vi "intersecAreaQuad.vi"(8 "error in (no error)":errorcluster, 9 "Ball/Enemy\nPosition":dbl[](array[numeric]), 10 "Game":refnum<class "Game.lvclass">, 11 "Utilities in":refnum<class "Utilities.lvclass">) -> (0 "error out":errorcluster, 2 "Pos de Interseção":dbl[](array[numeric]) format="%#_13g", 3 "Utilities out":refnum<class "Utilities.lvclass">)   [LabVIEW 2018, in "Utilities.lvclass"]
uses:
  Utilities.lvclass
  Game_class/Game.lvclass
  Game_class/Game.lvclass/Game.ctl
  Game_class/Read FieldRef.vi
  Field_class/Field.lvclass
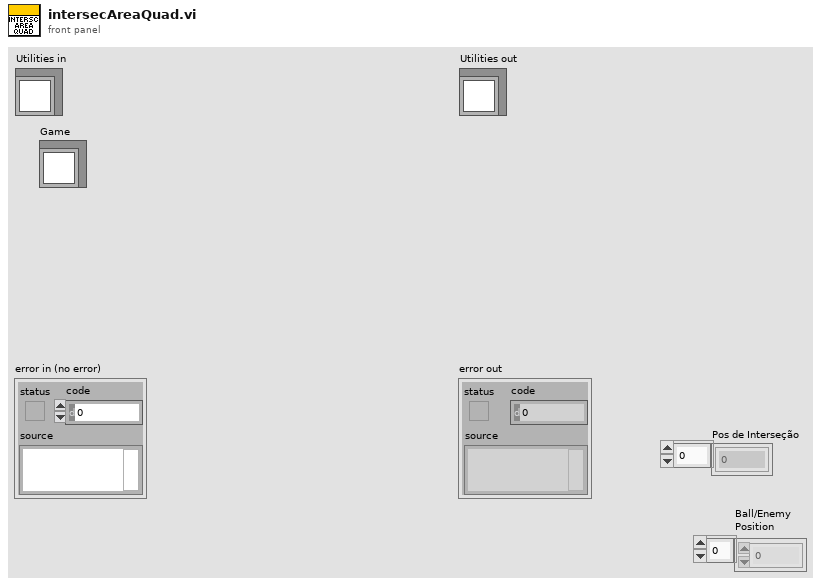
[diagram p1: front panel]
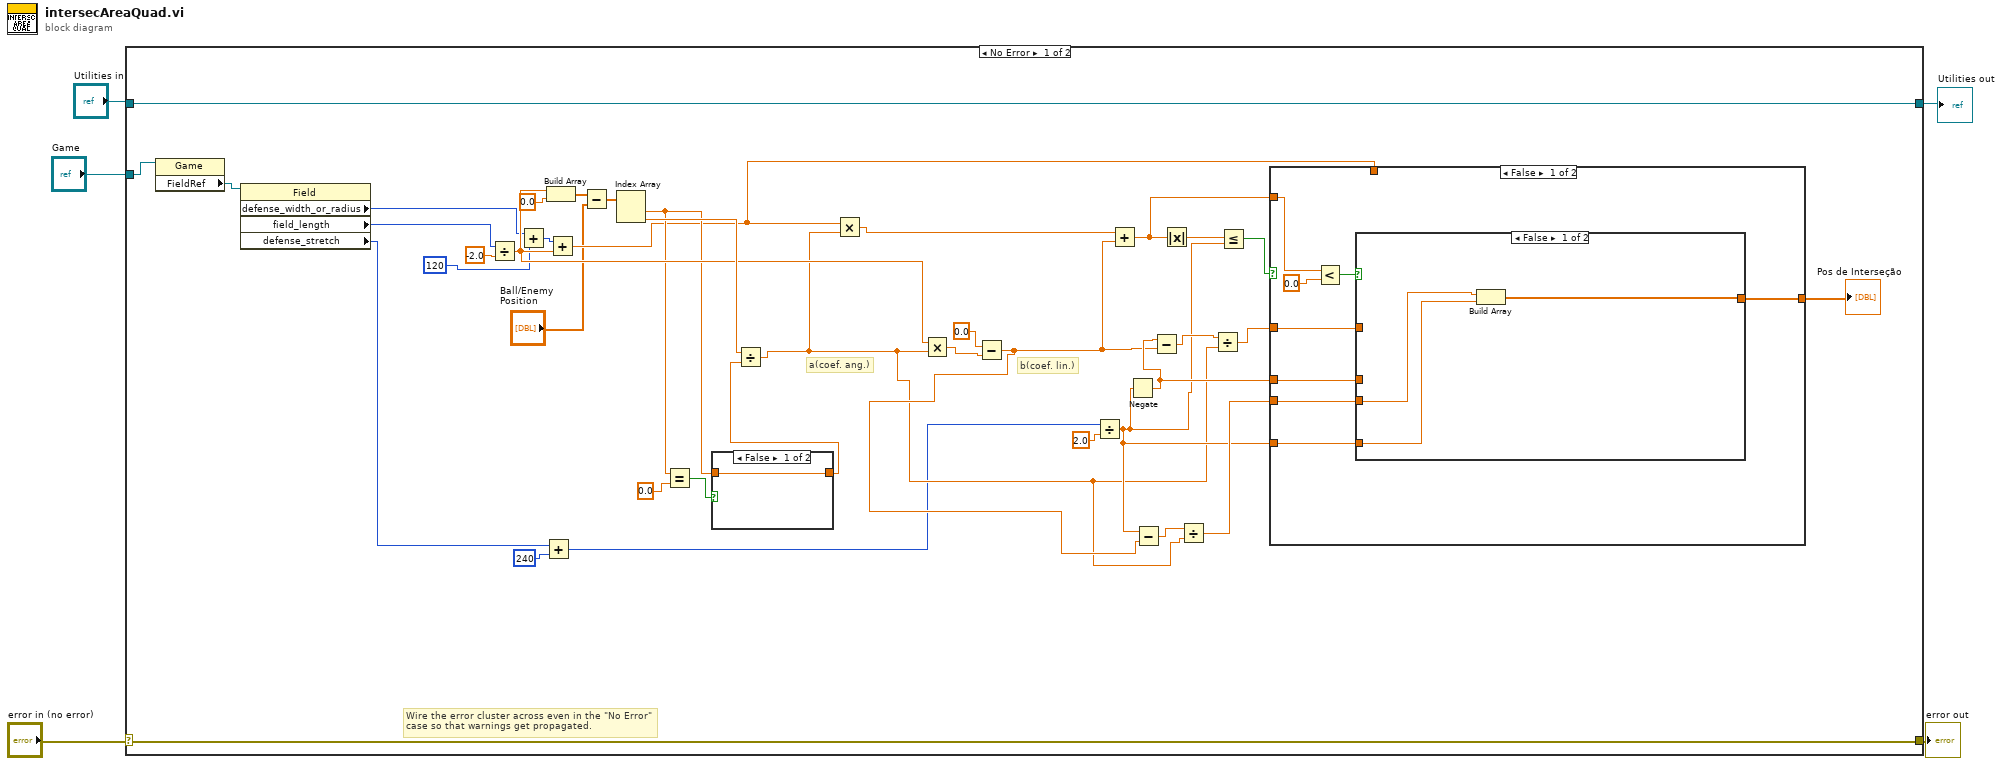
[diagram p0: block diagram]
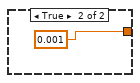
[diagram p2: hidden frame]
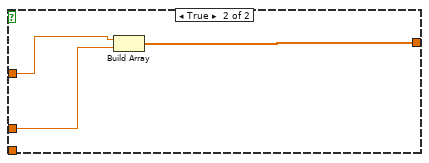
[diagram p3: hidden frame]
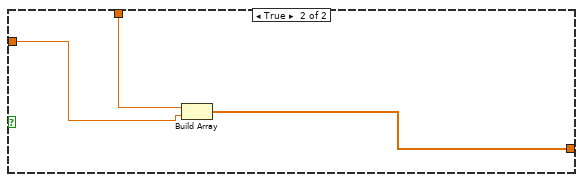
[diagram p4: hidden frame]
diagram:
  n1 = case shown="No Error" "error in (no error)" {
    selector: "error in (no error)" -> [w43 w65]
    tunnel: [w43 w65] -> w4
    tunnel: [w44 w64] -> w2
    tunnel: "Utilities in" -> [w44 w64]
    tunnel: "Game" -> [w11 _]
    frame No Error {
      # "b(coef. lin.)"
      # "a(coef. ang.)"
      # "Wire the error cluster across even in the \"No Error\"\ncase so that warnings get propagated."
      n2 = property class="Game"(reference=w11) -> ("FieldRef"=w10:refnum<class "Field.lvclass">)  [unwired: 1 in, 2 out]
      n3 = property class="Field"(reference=w10) -> ("defense_width_or_radius"=w9:i32, "field_length"=w8:i32, "defense_stretch"=w7:i32)  [unwired: 1 in, 2 out]
      n4 = Divide(x=w8, y=-2.0) -> (x/y=w35:dbl)
      n5 = Add(x=w9, y=u32 120) -> (x+y=w14:u32)
      n6 = Add(x=w7, y=u32 240) -> (x+y=w13:u32)
      n7 = Build Array(w35, 0.0 ("element")) -> (w40:dbl[])
      n8 = Add(x=w14, y=w35) -> (x+y=w16:dbl)
      n9 = Subtract(x=w40, y="Ball/Enemy\nPosition") -> (x-y=w39:dbl[])
      n10 = Index Array(array=w39) -> (element #1=w20:dbl, element #2=w38:dbl)  [unwired: 2 in]
      n11 = Equal?(x=w20, y=0.0) -> (x = y?=w21:bool)
      n12 = case shown="False" w21 {
        tunnel: w20 -> [w45 _]
        tunnel: [w45 0.001] -> w19
        frame False {
        }
        frame True {
        }
      }
      n13 = Divide(x=w38, y=w19) -> (x/y=w23:dbl)
      n14 = Multiply(x=w16, y=w23) -> (x*y=w34:dbl)
      n15 = Multiply(x=w35, y=w23) -> (x*y=w37:dbl)
      n16 = Subtract(x=0.0, y=w37) -> (x-y=w27:dbl)
      n17 = Divide(x=w13, y=2.0) -> (x/y=w24:dbl)
      n18 = Add(x=w34, y=w27) -> (x+y=w15:dbl)
      n19 = Negate(x=w24) -> (-x=w28:dbl)
      n20 = Subtract(x=w24, y=w27) -> (x-y=w26:dbl)
      n21 = Subtract(x=w28, y=w27) -> (x-y=w30:dbl)
      n22 = Absolute Value(x=w15) -> (abs(x)=w33:dbl)
      n23 = Divide(x=w26, y=w23) -> (x/y=w25:dbl)
      n24 = Divide(x=w30, y=w23) -> (x/y=w29:dbl)
      n25 = Less Or Equal?(x=w33, y=w24) -> (x <= y?=w31:bool)
      n26 = case shown="False" w31 {
        tunnel: w15 -> [w54 w61]
        tunnel: w16 -> [_ w62]
        tunnel: [w49 w63] -> w12
        tunnel: w29 -> [w51 _]
        tunnel: w28 -> [w50 _]
        tunnel: w25 -> [w48 _]
        tunnel: w24 -> [w47 _]
        frame False {
          n27 = Less?(x=w54, y=0.0) -> (x < y?=w52:bool)
          n28 = case shown="False" w52 {
            tunnel: w51 -> [_ w59]
            tunnel: w50 -> [_ w58]
            tunnel: [w57 w60] -> w49
            tunnel: w48 -> [w56 _]
            tunnel: w47 -> [w55 _]
            frame False {
              n29 = Build Array(w56, w55) -> (w57:dbl[])
            }
            frame True {
              n30 = Build Array(w59, w58) -> (w60:dbl[])
            }
          }
        }
        frame True {
          n31 = Build Array(w62, w61) -> (w63:dbl[])
        }
      }
      "Pos de Interseção" <- w12
    }
    frame Error {
    }
  }
  "error out" <- w4
  "Utilities out" <- w2
